vi "Fast Item Reference to Pointer FuncGlobal.vi"(5 "Action":enum16{"Open or Add", "Close Ref"}(ring), 8 "error in (no error)":errorcluster, 11 "Item Ref in":T2 format="%.0x") -> (0 "error out":errorcluster, 2 "Node Pointer":T1, 3 "Item Ref out":T2 format="%.0x", 4 "Found":bool)   [LabVIEW 2011]
uses:
  <vilib>/NI Veristand/Custom Device API/Custom Device Item Ref.ctl
  <vilib>/NI Veristand/Custom Device API/Custom Device Pointer.ctl
  NationalInstruments.VeriStand.SystemStorage
  <vilib>/NI Veristand/Custom Device API/Custom Device API.lvlib
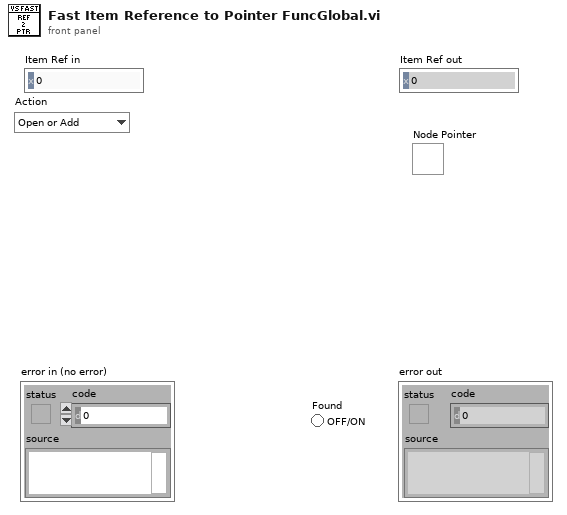
[diagram p1: front panel]
types:
  T1 = typedef "Custom Device API.lvlib/Custom Device Pointer.ctl" = refnum<k24>
  T2 = typedef "Custom Device API.lvlib/Custom Device Item Ref.ctl" = u64
  T3 = typedef "NIVS_DataStorage.lvlib/BaseNodeType.ctl" = refnum<k24>
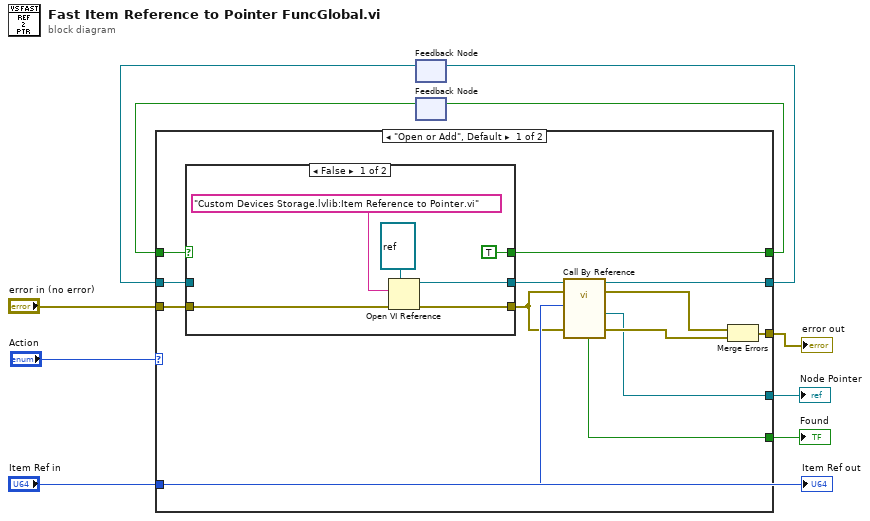
[diagram p0: block diagram]
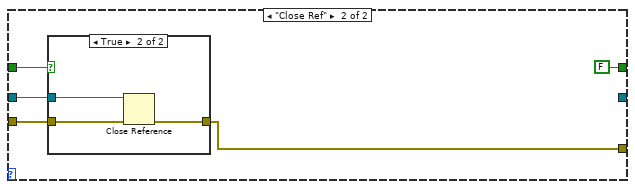
[diagram p3: hidden frame]
diagram:
  n1 = feedback #1() -> (w2:refnum<vi>)  [unwired: 1 in]
  n2 = feedback #2() -> (w3:bool)  [unwired: 1 in]
  n3 = case shown="\"Open or Add\", Default" "Action" {
    tunnel: [w22 w34] -> w10
    tunnel: "error in (no error)" -> [w21 w35]
    tunnel: "Item Ref in" -> [w20 _]
    tunnel: [w19 _] -> w7
    tunnel: [w18 _] -> w6
    tunnel: [w14 _] -> w5
    tunnel: [w13 FALSE] -> w4
    tunnel: w3 -> [w12 w37]
    tunnel: w2 -> [w11 w36]
    frame "Open or Add", Default {
      n4 = case shown="False" w12 {
        selector: w12 -> [_ w32]
        tunnel: w21 -> [w27 w30]
        tunnel: [w26 w30] -> w17
        tunnel: [w25 w31] -> w16
        tunnel: [TRUE w32] -> w13
        tunnel: w11 -> [_ w31]
        frame False {
          n5 = Open VI Reference(type specifier VI Refnum (for type only)=refnum<vi> refnum, vi path="Custom Devices Storage.lvlib:Item Reference to Pointer.vi", error in (no error)=w27) -> (vi reference=w25:refnum<vi>, error out=w26:errorcluster)  [unwired: 3 out]
        }
        frame True {
        }
      }
      n6 = call-by-ref "?"(reference=w16, error in=w17, 8:"error in (no error)"=w17, "Item Reference"=w20) -> (reference out=w14:refnum<vi>, error out=w15:errorcluster, 0:"error out"=w23:errorcluster, "FoundNode"=w18:T3, "Found"=w19:bool)  [unwired: 6 in, 1 out]
      n7 = Merge Errors(w15, w23) -> (w22:errorcluster)
    }
    frame "Close Ref" {
      n8 = case shown="True" w37 {
        tunnel: w36 -> [_ w41]
        tunnel: w35 -> [w38 w40]
        tunnel: [w38 w39] -> w34
        frame False {
        }
        frame True {
          n9 = Close Reference(reference=w41, error in (no error)=w40) -> (error out=w39:errorcluster)
        }
      }
    }
  }
  "error out" <- w10
  "Found" <- w7
  "Node Pointer" <- w6
  n10 = feedback-in #1(w5) -> ()
  n11 = feedback-in #2(w4) -> ()
  "Item Ref out" <- "Item Ref in"
